vi "Get Enum Type Specializations.vi"(8 "error in":errorcluster, 10 "measurement control path":path, 11 "measurement plugin service in":refnum<class "Measurement Plugin Service.lvclass">) -> (0 "error out":errorcluster, 2 "type specializations":T1[](array[typedef]), 3 "measurement plugin service out":refnum<class "Measurement Plugin Service.lvclass">)   [LabVIEW 2020, in "Measurement Plugin Measurement Server.lvlib"]
uses:
  Measurement Plugin Measurement Server.lvlib
  Measurement Plugin Service/Measurement Plugin Service.lvclass
  TypeDefs/Parameter Type Specialization.ctl
  TypeDefs/Type Specialization.ctl
  TypeDefs/Type Specialization Key.ctl
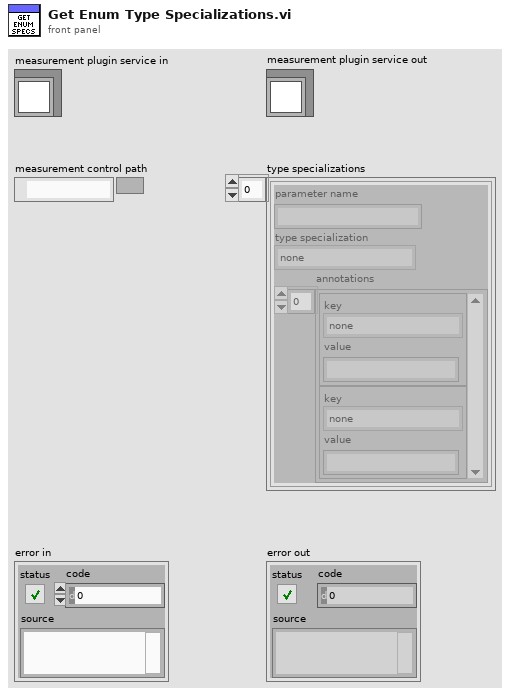
[diagram p1: front panel]
types:
  T1 = typedef "Measurement Plugin Measurement Server.lvlib/Parameter Type Specialization.ctl" = cluster{"parameter name":string, "type specialization":T2, "annotations":cluster{"key":T3, "value":string}[]}
  T2 = typedef "Measurement Plugin Measurement Server.lvlib/Type Specialization.ctl" = enum16{"none", "pin", "path", "enum", "ioresource"}
  T3 = typedef "Measurement Plugin Measurement Server.lvlib/Type Specialization Key.ctl" = enum16{"none", "pin.instrument_type", "enum.values", "ioresource.instrument_type"}
  T4 = cluster{"Enum reference out":refnum<vi>, "Label.Text":string}[]
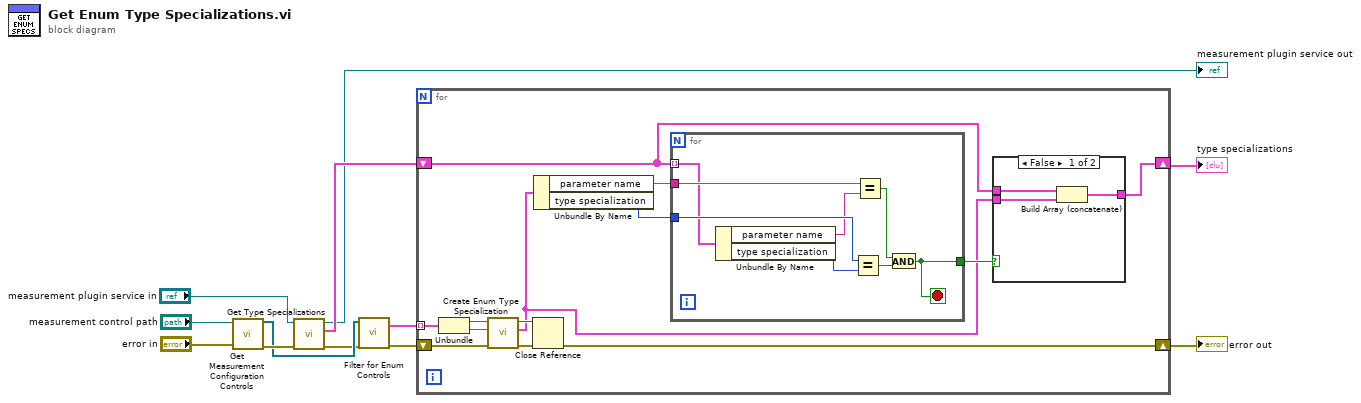
[diagram p0: block diagram]
diagram:
  n1 = call "Get Measurement Configuration Controls.vi"("error in"="error in", "measurement configuration control path"="measurement control path") -> ("error out"=w11:errorcluster, "controls"=w9:refnum<vi>[])  [unwired: 7 in]
  n2 = call-dynamic "Get Type Specializations.vi"("error in"=w11, "measurement plugin service in"="measurement plugin service in") -> ("error out"=w8:errorcluster, "type specializations"=w12:T1[], "measurement plugin service out"=→"measurement plugin service out":refnum<class "Measurement Plugin Service.lvclass">)  [unwired: 7 in]
  n3 = call "Filter for Enum Controls.vi"("error in"=w8, "controls"=w9) -> ("error out"=w10:errorcluster, "enum controls and labels"=w7:T4)  [unwired: 8 in]
  n4 = for {
    shift-right: [w20] -> w5
    shift-left: w10 -> [w16]
    tunnel: w7 -> [w15] mode=indexing
    shift-right: [w17] -> w6
    shift-left: w12 -> [w18]
    n5 = Unbundle(w15) -> ("Enum reference out"=w14:refnum<vi>, "Label.Text"=w13:string)
    n6 = call "Create Enum Type Specialization.vi"("error in"=w16, "parameter name"=w13, "enum reference in"=w14) -> ("error out"=w22:errorcluster, "parameter type specialization output"=w19:T1, "control reference out"=w21:refnum<vi>)  [unwired: 5 in]
    n7 = Close Reference(reference=w21, error in (no error)=w22) -> (error out=w20:errorcluster)
    n8 = Unbundle By Name(w19) -> ("parameter name"=w25:string, "type specialization"=w24:T2)
    n9 = for {
      tunnel: w25 -> [w35]
      tunnel: w24 -> [w36]
      tunnel: [w31] -> w23
      tunnel: w18 -> [w30] mode=indexing
      stop <- w31 stop-if-true
      n10 = Unbundle By Name(w30) -> ("parameter name"=w34:string, "type specialization"=w37:T2)
      n11 = Equal?(x=w36, y=w37) -> (x = y?=w32:bool)
      n12 = Equal?(x=w35, y=w34) -> (x = y?=w33:bool)
      n13 = And(x=w33, y=w32) -> (x .and. y?=w31:bool)
    }
    n14 = case shown="False" w23 {
      tunnel: w18 -> [w28 w29]
      tunnel: w19 -> [w26 _]
      tunnel: [w27 w29] -> w17
      frame False {
        n15 = Build Array (concatenate)(w28, w26) -> (w27:T1[])
      }
      frame True {
      }
    }
  }
  "type specializations" <- w6
  "error out" <- w5
